vi "RT Main.vi"() -> ()   [LabVIEW 2021]
doc: "Demonstrates the use of Transmission Control Protocol (TCP) to communicate between the host computer and one or multiple myRIO targets."
uses:
  <vilib>/myRIO/Express VI/Onboard Devices/LED/LED Express VI.xnode
  <vilib>/myRIO/Instrument Drivers/Onboard IO/DIO/vis/Write.vi
  <vilib>/myRIO/Instrument Drivers/Onboard IO/DIO/DIO.lvlib
  <vilib>/myRIO/Common/Instrument Driver Framework/myRIO v1.0/DIO/typedefs/DIO Channels Enum.ctl
  <vilib>/myRIO/Common/Instrument Driver Framework/myRIO v1.0/DIO/typedefs/DIO Channels List.ctl
  <vilib>/myRIO/Common/Instrument Driver Framework/Utilities/typedefs/Generic FPGA Reference.ctl
  <vilib>/myRIO/Common/Instrument Driver Framework/Utilities/typedefs/myRIO v1.0 Reference.ctl
  <vilib>/myRIO/Common/Instrument Driver Framework/Utilities/typedefs/Hardware Version Enum.ctl
  <vilib>/myRIO/Common/Instrument Driver Framework/Utilities/typedefs/myRIO Generic Hardware Reference.ctl
  <vilib>/myRIO/Instrument Drivers/Onboard IO/DIO/typedefs/DIO Reference.ctl
  <vilib>/myRIO/Instrument Drivers/Onboard IO/DIO/vis/myRIO DIO Open.xnode
  <vilib>/myRIO/Common/Instrument Driver Framework/Utilities/vis/Is FPGA Ref Available.vi
  <vilib>/myRIO/Instrument Drivers/Utilities/Utilities.lvlib
  <vilib>/myRIO/Common/Instrument Driver Framework/myRIO v1.0/DIO/vis/myRIO v1.2 Open DIO.vi
  <vilib>/userdefined/High Color/nirio_resource_hc.ctl
panel:
  out "LED Status":bool[](array[boolean])
  out "error out":errorcluster
  in  "Target Name":string="Target1"
  in  "Host IP Address":string="172.22.11.1"
  in  "Stop":bool
  # "Overview: Demonstrates the use of Transmission Control Protocol (TCP) to communicate between the host computer and one or multiple myRIO targets.\nInstructions:\n1. Ensure Desktop Main.vi is already running.\n2. Verify the value of Host IP Address. If it is incorrect, specify the correct value.\n3. Observe the LEDs on the myRIO device and the value of LED Status on this VI. They change when the value of LED on Desktop Main.vi changes.\n4. (Optional) To communicate with another myRIO target, create a new target, copy RT Main.vi, and add this VI under the new target. In the new RT Main.vi, specify a new name for Target Name.\n5. Click Stop to stop this VI. When you stop this VI, the value of Number of Client Connections on Desktop Main.vi changes."
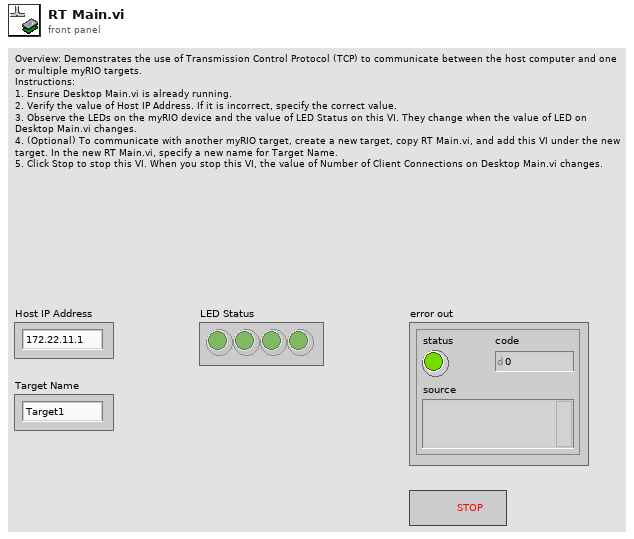
[diagram p1: front panel]
types:
  T1 = typedef "DIO.lvlib/DIO Reference.ctl" = cluster{"myRIO Reference":T2, "DIO Channels List":T6}
  T2 = typedef "myRIO Generic Hardware Reference.ctl" = cluster{"myRIO Model":T3, "myRIO Hardware Reference":T4}
  T3 = typedef "Hardware Version Enum.ctl" = enum16{"Unknown", "myRIO-1900", "myRIO-1950", "roboRIO", "NI ELVIS RIO CM", "ELVIS III"}
  T4 = typedef "myRIO v1.0 Reference.ctl" = cluster{"Generic FPGA Reference":T5, "Allow multiple opens":bool}
  T5 = typedef "Generic FPGA Reference.ctl" = refnum<k20>
  T6 = typedef "DIO Channels List.ctl" = T7[]
  T7 = typedef "DIO Channels Enum.ctl" = enum16{"Not Connected", "C/DIO0", "C/DIO1", "C/DIO2", "C/DIO3", "C/DIO4", "C/DIO5", "C/DIO6", "C/DIO7", "A/DIO0", "A/DIO1", "A/DIO2", "A/DIO3", "A/DIO4", "A/DIO5", "A/DIO6", "A/DIO7", "A/DIO8", "A/DIO9", "A/DIO10", "A/DIO11", "A/DIO12", "A/DIO13", "A/DIO14", "A/DIO15", "A/DIO16", "A/DIO17", "A/DIO18", "A/DIO19", "B/DIO0", "B/DIO1", "B/DIO2", "B/DIO3", "B/DIO4", "B/DIO5", "B/DIO6", "B/DIO7", "B/DIO8", "B/DIO9", "B/DIO10", "B/DIO11", "B/DIO12", "B/DIO13", "B/DIO14", "B/DIO15", "B/DIO16", "B/DIO17", "B/DIO18", "B/DIO19", "LED0", "LED1", "LED2", "LED3", "Button0", "DIO/DIO0", "DIO/DIO1", "DIO/DIO2", "DIO/DIO3", "DIO/DIO4", "DIO/DIO5", "DIO/DIO6", "DIO/DIO7", "DIO/DIO8", "DIO/DIO9", "SPI/CS0", "SPI/CS1", "SPI/CS2", "SPI/CS3", "LED RADIO (Green)", "LED RADIO (Red)", "LED COMM (Green)", "LED COMM (Red)", "LED MODE (Green)", "LED MODE (Red)"}
  T8 = typedef "nirio_resource_hc.ctl" = tag
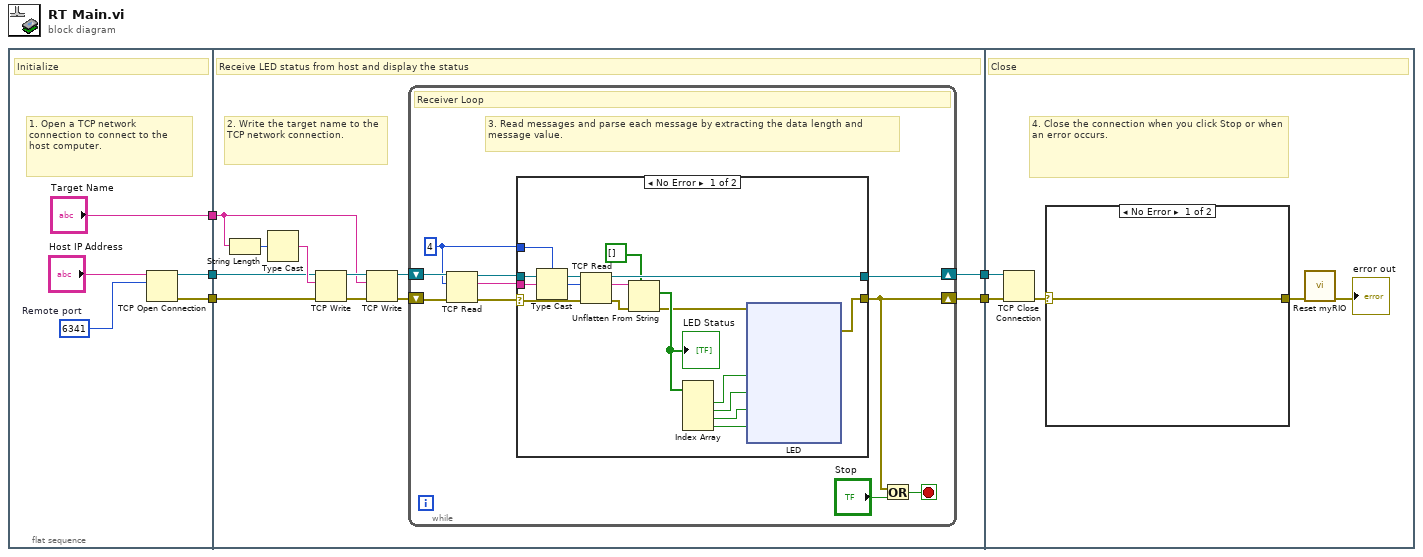
[diagram p0: block diagram]
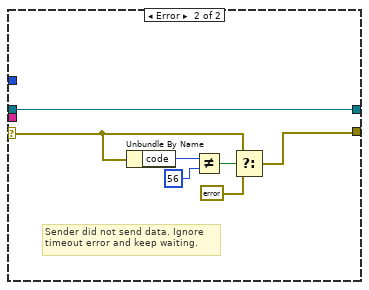
[diagram p2: hidden frame]
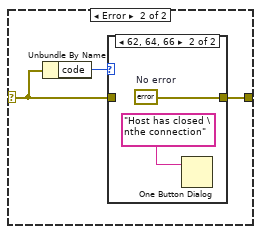
[diagram p3: hidden frame]
diagram:
  n1 = flat-sequence {
    tunnel: [w8] -> w5
    tunnel: [w7] -> w4
    tunnel: ["Target Name"] -> w3
    tunnel: w5 -> [w13]
    tunnel: w4 -> [w12]
    tunnel: w3 -> [w11]
    tunnel: [w15] -> w2
    tunnel: [w14] -> w1
    tunnel: w2 -> [w96]
    tunnel: w1 -> [w97]
    frame #0 {
      w10 = u16 6341  # Remote port
      # "1. Open a TCP network connection to connect to the host computer."
      # "Initialize"
      n2 = TCP Open Connection(address="Host IP Address", remote port or service name=w10) -> (connection ID=w7:refnum<k5>, error out=w8:errorcluster)  [unwired: 3 in]
    }
    frame #1 {
      # "2. Write the target name to the TCP network connection."
      # "Receive LED status from host and display the status"
      n3 = String Length(string=w11) -> (length=w17:i32)
      n4 = Type Cast(x=w17) -> (*(type *) &x=w16:string)  [unwired: 1 in]
      n5 = TCP Write(connection ID=w12, data in=w16, error in (no error)=w13) -> (connection ID out=w19:refnum<k5>, error out=w21:errorcluster)  [unwired: 1 in, 1 out]
      n6 = TCP Write(connection ID=w19, data in=w11, error in (no error)=w21) -> (connection ID out=w20:refnum<k5>, error out=w18:errorcluster)  [unwired: 1 in, 1 out]
      n7 = while {
        shift-right: [w22] -> w14
        shift-left: w20 -> [w29]
        shift-right: [w23] -> w15
        shift-left: w18 -> [w28]
        stop <- w30 stop-if-true
        w24 = 4 ("bytes to read")
        # "3. Read messages and parse each message by extracting the data length and message value."
        # "Receiver Loop"
        n8 = TCP Read(connection ID=w29, bytes to read=w24, error in (no error)=w28) -> (connection ID out=w27:refnum<k5>, data out=w25:string, error out=w26:errorcluster)  [unwired: 2 in]
        n9 = case shown="No Error" w26 {
          selector: w26 -> [w34 w86]
          tunnel: w25 -> [w47 _]
          tunnel: w24 -> [w46 _]
          tunnel: w27 -> [w44 w92]
          tunnel: [w41 w92] -> w22
          tunnel: [w33 w87] -> w23
          frame No Error {
            n10 = Type Cast(type=w46, x=w47) -> (*(type *) &x=w45:i32)
            n11 = TCP Read(connection ID=w44, bytes to read=w45, error in (no error)=w34) -> (connection ID out=w41:refnum<k5>, data out=w43:string, error out=w42:errorcluster)  [unwired: 2 in]
            n12 = Unflatten From String(type=bool[] [], binary string=w43, error in (no error)=w42) -> (value=w39:bool[], error out=w32:errorcluster)  [unwired: 2 in, 1 out]
            "LED Status" <- w39
            n13 = Index Array(array=w39) -> (element #1=w38:bool, element #2=w37:bool, element #3=w36:bool, element #4=w35:bool)  [unwired: 4 in]
            n14 = xnode "LED"("LED0"=w38, "LED1"=w37, "LED2"=w36, "LED3"=w35, "error in (no error)"=w32) -> ("error out"=w33:errorcluster)
          }
          frame Error {
            # "Sender did not send data. Ignore \ntimeout error and keep waiting."
            n15 = Unbundle By Name(w86) -> ("code"=w89:i32)
            n16 = Not Equal?(x=w89, y=56) -> (x != y?=w88:bool)
            n17 = Select(t=w86, s=w88, f=errorcluster {"status"=FALSE, "code"=0, "source"=""} ("error out")) -> (s? t:f=w87:errorcluster)
          }
        }
        n18 = Or(x=w23, y="Stop") -> (x .or. y?=w30:bool)
      }
    }
    frame #2 {
      # "4. Close the connection when you click Stop or when an error occurs."
      # "Close"
      n19 = TCP Close Connection(connection ID=w97, error in (no error)=w96) -> (error out=w94:errorcluster)  [unwired: 1 in, 1 out]
      n20 = case shown="No Error" w94 {
        selector: w94 -> [w98 w99]
        tunnel: [w98 w100] -> w93
        frame No Error {
        }
        frame Error {
          n21 = Unbundle By Name(w99) -> ("code"=w101:i32)
          n22 = case shown="62, 64, 66" w101 {
            tunnel: w99 -> [w102 _]
            tunnel: [w102 w103] -> w100
            frame Default {
            }
            frame 62, 64, 66 {
              w103 = errorcluster {"status"=FALSE, "code"=0, "source"=""}  # No error
              n23 = One Button Dialog(message="Host has closed \nthe connection") -> ()  [unwired: 1 in, 1 out]
            }
          }
        }
      }
      n24 = call <vilib>:"Reset myRIO.vi"("error in (no error)"=w93) -> ("error out"=→"error out":errorcluster)  [unwired: 10 in]
    }
  }
